vi "Array_2.vi"() -> ()   [LabVIEW 2023]
panel:
  out "appended array 3":string[](array[string])
  out "appended array 2":string[][](array[string])
  out "appended array":string[](array[string])
  in  "Array 2":string[](array[string])
  in  "Array":string[](array[string])
  in  "String":string
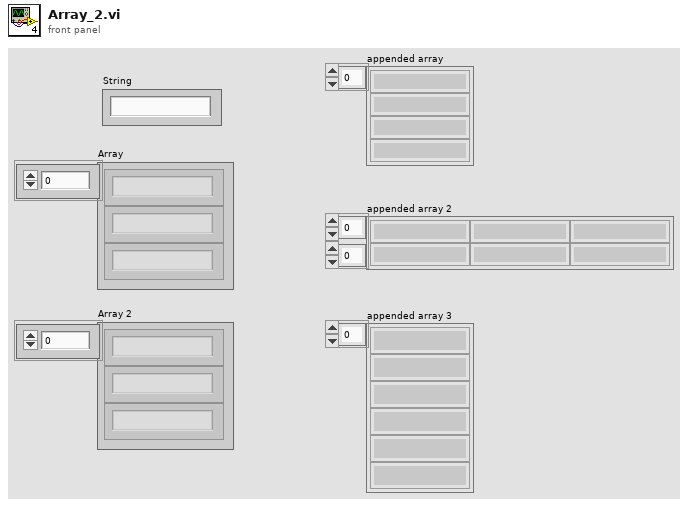
[diagram p1: front panel]
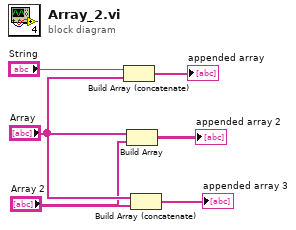
[diagram p0: block diagram]
diagram:
  n1 = Build Array (concatenate)("String", "Array") -> (→"appended array":string[])
  n2 = Build Array("Array", "Array 2") -> (→"appended array 2":string[][])
  n3 = Build Array (concatenate)("Array", "Array 2") -> (→"appended array 3":string[])
